vi "Example of default load and save.vi"() -> ()   [LabVIEW 2020]
uses:
  Default contorls manipulator.lvclass
panel:
  out "Path to the configuration file":path
  in  "Stop":bool
  in  "The test String":string
  in  "The test Boolean":bool
  in  "The test Numeric":dbl
  # "Intro: \nTry to modified values of the control after VI stopped. \nThese controls will be load after VI run."
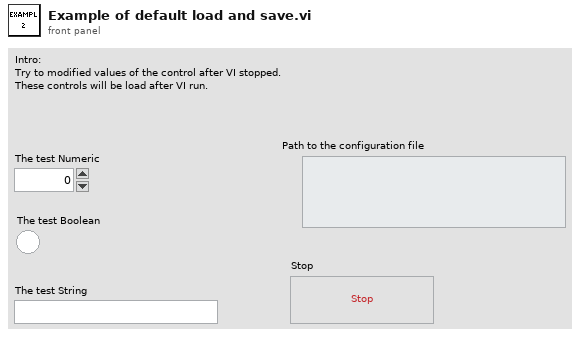
[diagram p1: front panel]
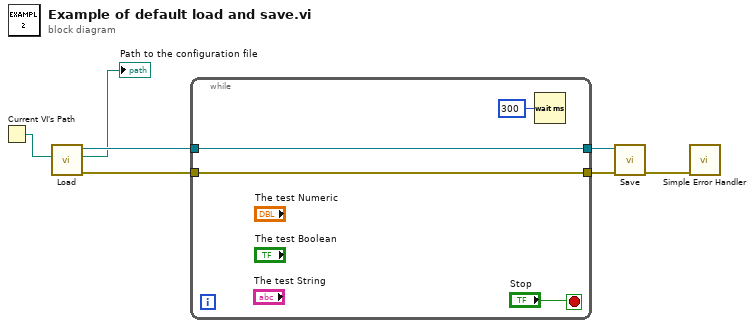
[diagram p0: block diagram]
diagram:
  n1 = Current VI's Path() -> (path=w7:path)
  n2 = call "Load.vi"("VI path"=w7) -> ("error out"=w3:errorcluster, "Configuration file path (*.ini)"=→"Path to the configuration file":path, "Default contorls manipulator out"=w5:refnum<class "Default contorls manipulator.lvclass">)  [unwired: 8 in]
  n3 = while {
    tunnel: [w11] -> w6
    tunnel: w5 -> [w11]
    tunnel: [w10] -> w4
    tunnel: w3 -> [w10]
    stop <- "Stop" stop-if-true
    n4 = Wait (ms)(milliseconds to wait=u32 300) -> ()  [unwired: 1 out]
  }
  n5 = call "Save.vi"("error in (no error)"=w4, "Default contorls manipulator in"=w6) -> ("error out"=w2:errorcluster)  [unwired: 6 in, 3 out]
  n6 = call <vilib>:"Simple Error Handler.vi"("error in (no error)"=w2) -> ()  [unwired: 4 in, 5 out]
